vi "execute.vi"(8 "error in (no error)":errorcluster, 10 "Context in":refnum<class "Context.lvclass">, 11 "EnterControlCommand in":refnum<class "EnterControlCommand.lvclass">) -> (0 "error out":errorcluster, 2 "Context out":refnum<class "Context.lvclass">, 3 "EnterControlCommand out":refnum<class "EnterControlCommand.lvclass">)   [LabVIEW 2016, in "EnterControlCommand.lvclass"]
uses:
  EnterControlCommand.lvclass
  Context/Context/Context.lvclass
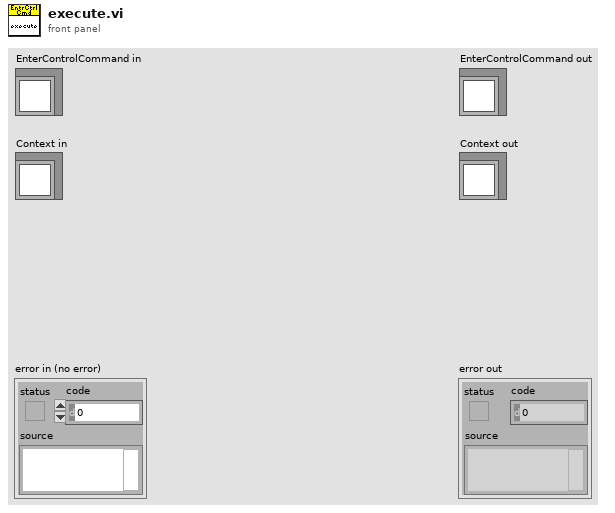
[diagram p1: front panel]
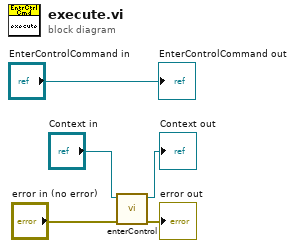
[diagram p0: block diagram]
diagram:
  n1 = call-dynamic "enterControl.vi"("error in (no error)"="error in (no error)", "Context in"="Context in") -> ("error out"=→"error out":errorcluster, "Context out"=→"Context out":refnum<class "Context.lvclass">)  [unwired: 8 in]
  "EnterControlCommand out" <- "EnterControlCommand in"
